vi "Write Configuration File.vi"(8 "error in (no error)":errorcluster, 11 "Inst.MOTOR in":refnum<class "Inst.MOTOR.lvclass">) -> (0 "error out":errorcluster, 3 "Inst.MOTOR out":refnum<class "Inst.MOTOR.lvclass">)   [LabVIEW 2019, in "Inst.MOTOR.lvclass"]
uses:
  Inst.MOTOR.lvclass
  C:/Program Files (x86)/National Instruments/LabVIEW 2019/user.lib/LevyLab/Instrument Framework/SMOs/Instrument/Instrument.lvclass
  Inst.MOTOR.lvclass/Inst.MOTOR.ctl
  <userlib>/LevyLab/Instrument Framework/SMOs/Instrument/Instrument.lvclass/Instrument.ctl
  <userlib>/Levylab/Instrument Framework/SMOs/Configuration/Configuration.lvclass/Configuration.ctl
  <userlib>/Levylab/Instrument Framework/SMOs/Configuration/Write Section.vi
  <userlib>/LevyLab/Instrument Framework/SMOs/Instrument/Instrument.lvclass
  C:/Program Files (x86)/National Instruments/LabVIEW 2019/vi.lib/JKI/JKI SMO/SMO/SMO.lvclass
  <vilib>/JKI/JKI SMO/SMO/Protected/ThisLevelClassName.vi
  <userlib>/Levylab/Instrument Framework/Instrument Types/VSource/Instrument.VSource.lvclass
  <userlib>/Levylab/Instrument Framework/SMOs/Configuration/Configuration.lvclass
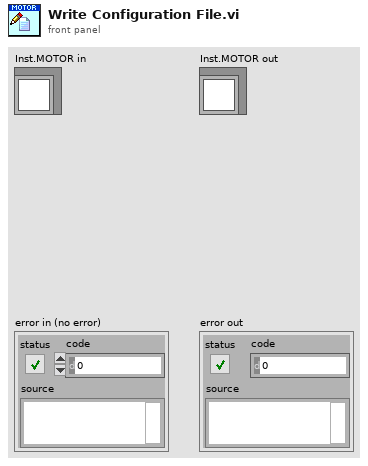
[diagram p1: front panel]
types:
  T1 = typedef "Inst.MOTOR.lvclass/Inst.MOTOR.Configuration--Cluster.ctl" = cluster{"Example Setting 1":dbl, "Example Setting 2":dbl, "Example Setting 3":string}
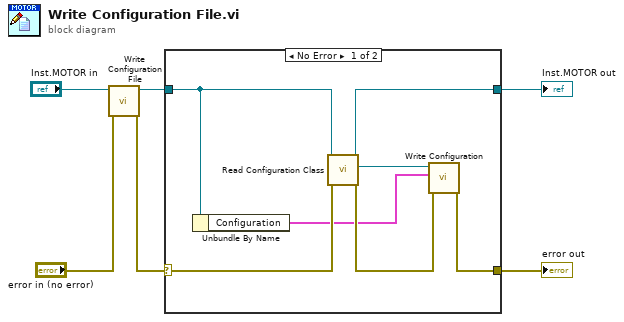
[diagram p0: block diagram]
diagram:
  n1 = call-parent "Write Configuration File.vi"("error in (no error)"="error in (no error)", "Instrument in"="Inst.MOTOR in") -> ("error out"=w3:errorcluster, "Instrument out"=w1:refnum<class "Inst.MOTOR.lvclass">)  [unwired: 8 in]
  n2 = case shown="No Error" w3 {
    selector: w3 -> [w9 w15]
    tunnel: w1 -> [w8 w14]
    tunnel: [w12 w14] -> w6
    tunnel: [w11 w15] -> w5
    frame No Error {
      n3 = Unbundle By Name(w8) -> ("Configuration"=w7:T1)
      n4 = call <userlib>:"Read Configuration Class.vi"("error in (no error)"=w9, "Instrument in"=w8) -> ("error out"=w13:errorcluster, "Configuration"=w10:refnum<class "Configuration.lvclass">, "Instrument out"=w12:refnum<class "Inst.MOTOR.lvclass">)  [unwired: 7 in]
      n5 = call <userlib>:"Write Configuration.vi"("error in (no error)"=w13, "Variant"=w7, "Configuration in"=w10) -> ("error out"=w11:errorcluster)  [unwired: 7 in, 1 out]
    }
    frame Error {
    }
  }
  "Inst.MOTOR out" <- w6
  "error out" <- w5
